vi "Untitled 3.vi"() -> ()   [LabVIEW 2016]
uses:
  Stanford Research 830.lvlib
panel:
  in  "VISA resource name":refnum<visa-resource-name>
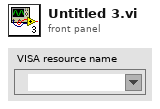
[diagram p1: front panel]
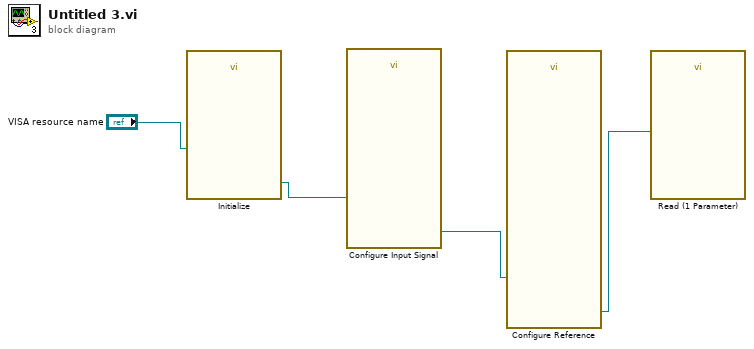
[diagram p0: block diagram]
diagram:
  n1 = call "Initialize.vi"("VISA resource name"="VISA resource name") -> ("VISA resource name out"=w3:refnum<visa-resource-name>)  [unwired: 9 in, 1 out]
  n2 = call "Configure Input Signal.vi"("VISA resource name"=w3) -> ("VISA resource name out"=w2:refnum<visa-resource-name>)  [unwired: 9 in, 1 out]
  n3 = call "Configure Reference.vi"("VISA resource name"=w2) -> ("VISA resource name out"=w1:refnum<visa-resource-name>)  [unwired: 13 in, 1 out]
  n4 = call "Read (1 Parameter).vi"("VISA resource name"=w1) -> ()  [unwired: 8 in, 3 out]
